vi "Launch New Task.vi"(8 "error in (no error)":errorcluster, 9 "Promise":refnum<class "Promise.lvclass">, 10 "Task":refnum<class "Task.lvclass">, 11 "VolatusCore in":refnum<class "VolatusCore.lvclass">) -> (0 "error out":errorcluster, 3 "VolatusCore out":refnum<class "VolatusCore.lvclass">)   [LabVIEW 2020, in "Volatus.lvlib" / "VolatusCore.lvclass"]
uses:
  VolatusCore.lvclass
  Task/Task.lvclass
  lv-promises/Promises/Promise/Promise.lvclass
  TaskEnQrValue/TaskEnQrValue.lvclass/TaskEnQrValue.ctl
  TaskEnQrValue/TaskEnQrValue.lvclass
  C:/dev/lv20CE/relink/lv-promises/Promises/Value/Value.lvclass
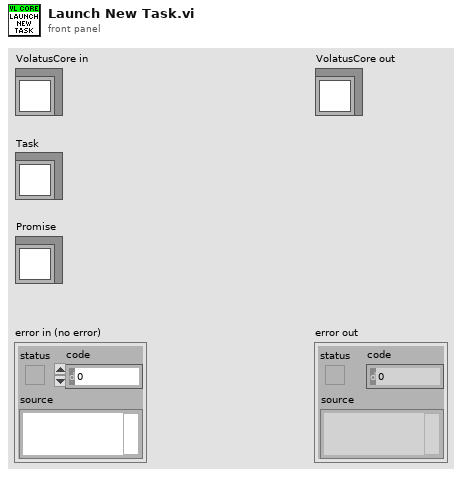
[diagram p1: front panel]
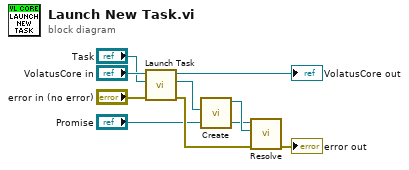
[diagram p0: block diagram]
diagram:
  n1 = call "Launch Task.vi"("error in (no error)"="error in (no error)", "Task"="Task", "VolatusCore in"="VolatusCore in") -> ("error out"=w9:errorcluster, "EnQr"=w3:refnum<class "Message Enqueuer.lvclass">, "VolatusCore out"=→"VolatusCore out":refnum<class "VolatusCore.lvclass">)  [unwired: 6 in]
  n2 = call "Create.vi"("EnQr"=w3) -> ("TaskEnQrValue out"=w4:refnum<class "TaskEnQrValue.lvclass">)  [unwired: 10 in]
  n3 = call "Resolve.vi"("error in (no error)"=w9, "Result"=w4, "Promise in"="Promise") -> ("error out"=→"error out":errorcluster)  [unwired: 7 in, 1 out]
